vi "Bit Pack.vi"(11 "Values":bool[](array[boolean])) -> (3 "Packed Values":u8[](array[numeric]))   [LabVIEW 2020, in "Device.lvlib"]
uses:
  Device.lvlib
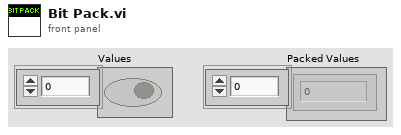
[diagram p1: front panel]
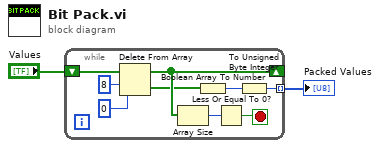
[diagram p0: block diagram]
diagram:
  n1 = while {
    shift-right: [w8] -> _
    shift-left: "Values" -> [w11]
    tunnel: [w3] -> w1 mode=indexing
    stop <- w6 stop-if-true
    n2 = Delete From Array(array=w11, length=8 ("index"), index=0 ("length")) -> (deleted portion=w5:bool[], array with subset deleted=w8:bool[])
    n3 = Array Size(array=w8) -> (size(s)=w7:i32)
    n4 = Boolean Array To Number(Boolean array=w5) -> (number=w4:u32)
    n5 = Less Or Equal To 0?(x=w7) -> (x <= 0?=w6:bool)
    n6 = To Unsigned Byte Integer(number=w4) -> (unsigned 8bit integer=w3:u8)
  }
  "Packed Values" <- w1
